vi "UIRef.vi"(8 "error in":errorcluster, 11 "EngineTags in":refnum<class "Engine Mappings.lvclass">) -> (0 "error out":errorcluster, 2 "VI refnum":refnum<vi>, 3 "EngineTags out":refnum<class "Engine Mappings.lvclass">)   [LabVIEW 2013, in "PL Framework Configuration Tool.lvlib" / "Engine Mappings.lvclass"]
uses:
  Engine Mappings.lvclass
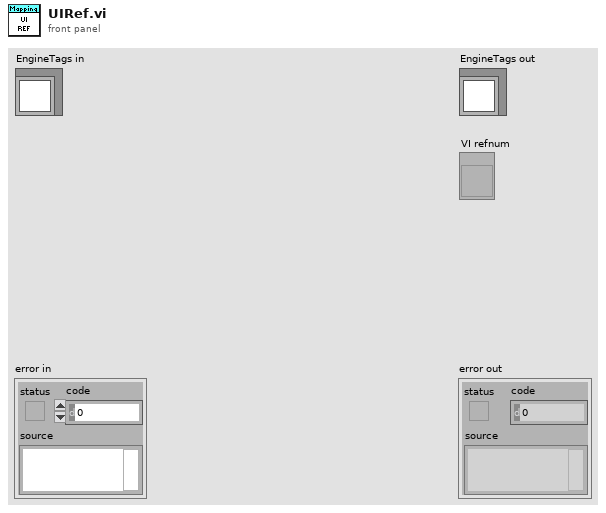
[diagram p1: front panel]
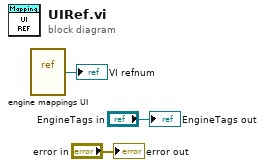
[diagram p0: block diagram]
diagram:
  n1 = vi-ref "engine mappings UI.vi"() -> (→"VI refnum":refnum<vi>)
  "error out" <- "error in"
  "EngineTags out" <- "EngineTags in"
